vi "peg-in-hole Test with ref.vi"() -> ()   [LabVIEW 2013]
uses:
  Arm Globals.vi
  <vilib>/Utility/file.llb/Write To Spreadsheet File (DBL).vi
panel:
  in  "Pin Array":dbl[](array[numeric])
  in  "Save":bool
  in  "Peg Positions":i32[](array[numeric])
  out "Loops Remaining":i32=1
  out "Peg":i32=1
  out "Times":dbl[](array[numeric])=[14.65, 8.4, 8.4, 7.7, 7.75, 7.5, 8.1, 7.7, 8.4, 7.65, 7.65, 7.7, 8.35, 7.7, 32.2, 8.1, 8.25, 7.5, 7.8, 7.8, 7.7, 7.8500000000000005, 8.5, 7.4, 8.85, 8.05, 8.55, 7.5, 8.2, 7.8, 8.8, 7.55, 8.25, 7.3500000000000005, 8.85, 7.5, 8.65, 7.65, 8.950000000000001, 7.7, 7.5, 14.85, 7.6000000000000005, 7.6000000000000005, 9.05, 14.15, 15.200000000000001, 7.6000000000000005, 15.4, 7.5, 17.45, 7.5, 35.6, 7.75, 22.45, 7.45, 8.9, 7.75, 23.150000000000002, 7.95, 7.6000000000000005, 8.5, 8.9, 7.95, 8.2, 47.099000000000004, 21.150000000000002, 71.75, 9.0, 7.8500000000000005, 43.7, 16.1, 8.2, 8.1, 8.700000000000001, 16.2, 8.700000000000001, 7.7, 15.450000000000001, 7.3500000000000005, 7.8500000000000005, 7.55, 14.4, 7.4, 8.3, 7.6000000000000005, 14.4, 7.75, 8.3, 7.7, 8.25, 7.75, 8.0, 7.45, 14.3, 7.5, 8.2, 7.4, 7.7490000000000006, 7.8, 8.15, 7.5, 7.7, 7.7]
  out "Status":string="Test.4"
  in  "Stop":bool
  out "error out":errorcluster
  # "1\n2\n3\n4\n5\n6\n7"
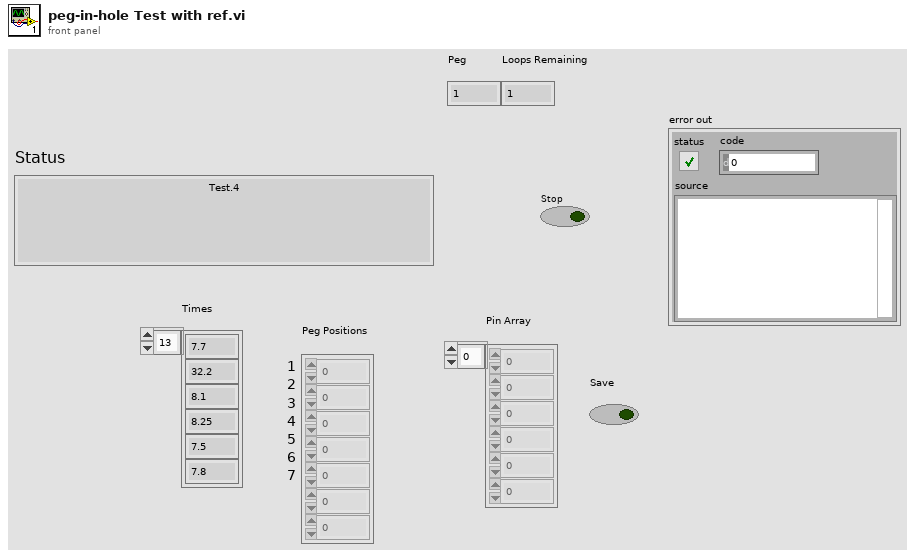
[diagram p1: front panel]
types:
  T1 = cluster{"X":dbl, "Y":dbl, "Z":dbl, "O":dbl, "A":dbl, "T":dbl}
  T2 = cluster{"X":dbl, "Y":dbl, "Z":dbl, "O":dbl, "A":dbl, "T":dbl}[]
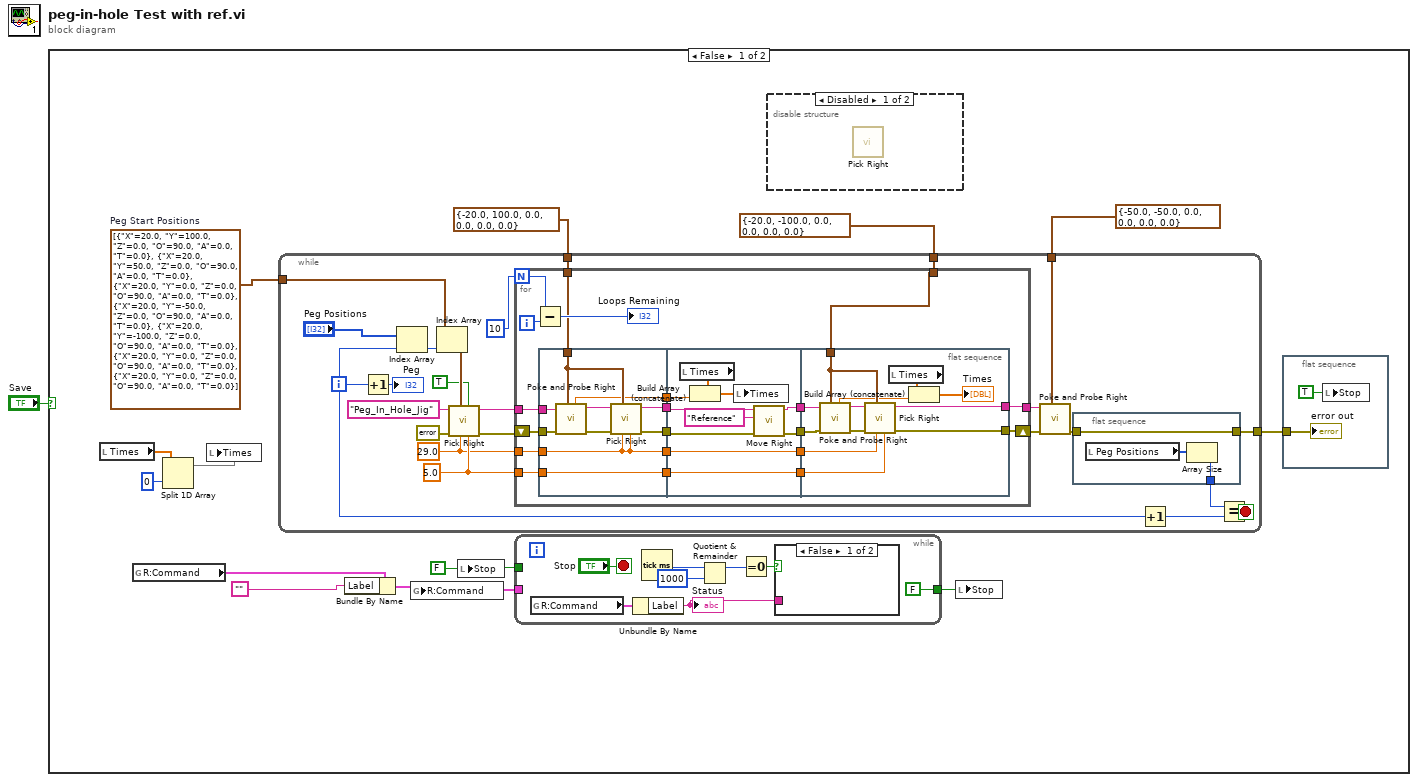
[diagram p0: block diagram]
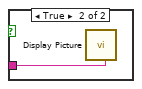
[diagram p3: hidden frame]
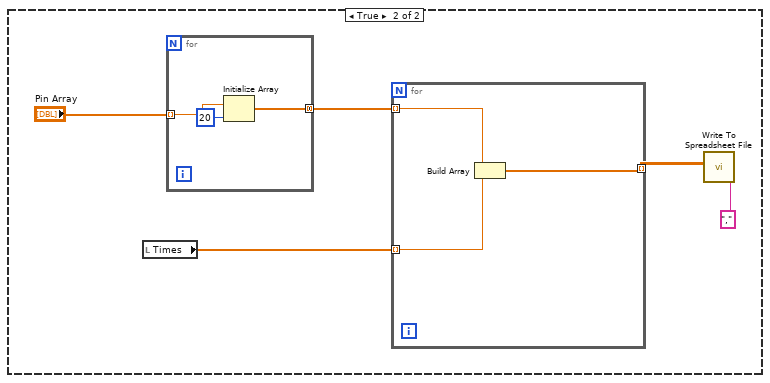
[diagram p4: hidden frame]
diagram:
  n1 = case shown="False" "Save" {
    frame False {
      w10 = FALSE ("Stop")
      w5 = T2 [{"X"=20.0, "Y"=100.0, "Z"=0.0, "O"=90.0, "A"=0.0, "T"=0.0}, {"X"=20.0, "Y"=50.0, "Z"=0.0, "O"=90.0, "A"=0.0, "T"=0.0}, {"X"=20.0, "Y"=0.0, "Z"=0.0, "O"=90.0, "A"=0.0, "T"=0.0}, {"X"=20.0, "Y"=-50.0, "Z"=0.0, "O"=90.0, "A"=0.0, "T"=0.0}, {"X"=20.0, "Y"=-100.0, "Z"=0.0, "O"=90.0, "A"=0.0, "T"=0.0}, {"X"=20.0, "Y"=0.0, "Z"=0.0, "O"=90.0, "A"=0.0, "T"=0.0}, {"X"=20.0, "Y"=0.0, "Z"=0.0, "O"=90.0, "A"=0.0, "T"=0.0}]  # Peg Start Positions
      n2 = local read "Times"() -> (w13:dbl[])
      n3 = global read "Arm Globals.vi" "R:Command"() -> (w6:cluster{"Label":string, "Angles":dbl[]})
      n4 = Split 1D Array(array=w13, index=0) -> (first subarray=w11:dbl[])  [unwired: 1 out]
      n5 = local write "Times"(w11) -> ()
      n6 = while {
        tunnel: [w21] -> w14
        tunnel: w5 -> [w34]
        tunnel: T1 {"X"=-20.0, "Y"=-100.0, "Z"=0.0, "O"=0.0, "A"=0.0, "T"=0.0} ("x") -> [w35]
        tunnel: T1 {"X"=-50.0, "Y"=-50.0, "Z"=0.0, "O"=0.0, "A"=0.0, "T"=0.0} ("x") -> [w36]
        tunnel: T1 {"X"=-20.0, "Y"=100.0, "Z"=0.0, "O"=0.0, "A"=0.0, "T"=0.0} ("x") -> [w29]
        i -> [w16]
        stop <- w26 stop-if-true
        w18 = sgl 5.0 ("Threshold")
        w17 = sgl 29.0 ("Target Position")
        n7 = Increment(x=w16) -> (x+1=→"Peg":i32)
        n8 = Index Array(array="Peg Positions", index=w16) -> (element=w32:i32)
        n9 = Index Array(array=w34, index=w32) -> (element=w33:T1)
        n10 = call "Pick Right.vi"("Threshold"=w18, "Pause on Miss?"=TRUE, "Target Position"=w17, "Pick"=w33, "error in"=errorcluster {"status"=FALSE, "code"=0, "source"=""}, "Location"="Peg_In_Hole_Jig") -> ("error out"=w31:errorcluster, "Location Out"=w24:string)  [unwired: 4 in]
        n11 = for {
          N: 10 -> [w61]
          shift-right: [w50] -> w30
          shift-left: w31 -> [w58]
          tunnel: w35 -> [w51]
          tunnel: w29 -> [w56]
          tunnel: w24 -> [w57]
          tunnel: [w49] -> w23
          tunnel: w18 -> [w45]
          tunnel: w17 -> [w42]
          i -> [w60]
          n12 = Subtract(x=w61, y=w60) -> (x-y=→"Loops Remaining":i32)
          n13 = flat-sequence {
            tunnel: w58 -> [w71]
            tunnel: w57 -> [w70]
            tunnel: w56 -> [w69]
            tunnel: [w67] -> w55
            tunnel: [w65] -> w54
            tunnel: [w64] -> w53
            tunnel: [w63] -> w46
            tunnel: w45 -> [w63]
            tunnel: [w62] -> w43
            tunnel: w42 -> [w62]
            tunnel: w55 -> [w77]
            tunnel: w54 -> [w80]
            tunnel: w53 -> [w76]
            tunnel: [w78] -> w52
            tunnel: [w75] -> w48
            tunnel: [w73] -> w47
            tunnel: w46 -> [w73]
            tunnel: [w72] -> w44
            tunnel: w43 -> [w72]
            tunnel: w52 -> [w92]
            tunnel: w51 -> [w89]
            tunnel: [w85] -> w50
            tunnel: [w84] -> w49
            tunnel: w48 -> [w93]
            tunnel: w47 -> [w83]
            tunnel: w44 -> [w82]
            frame #0 {
              n14 = call "Poke and Probe Right.vi"("Goal"=w69, "error in"=w71, "Location"=w70) -> ("error out"=w66:errorcluster, "Location Out"=w68:string, "time"=w65:dbl)  [unwired: 6 in]
              n15 = call "Pick Right.vi"("Threshold"=w62, "Target Position"=w62, "Pick"=w69, "error in"=w66, "Location"=w68) -> ("error out"=w67:errorcluster, "Location Out"=w64:string)  [unwired: 5 in]
            }
            frame #1 {
              n16 = local read "Times"() -> (w81:dbl[])
              n17 = Build Array (concatenate)(w81, w80) -> (w79:dbl[])
              n18 = local write "Times"(w79) -> ()
              n19 = call "Move Right.vi"("error in"=w77, "Mask"="Reference", "Location"=w76) -> ("error out"=w78:errorcluster, "Location Out"=w75:string)  [unwired: 4 in, 3 out]
            }
            frame #2 {
              n20 = call "Poke and Probe Right.vi"("Goal"=w89, "error in"=w92, "Location"=w93) -> ("error out"=w91:errorcluster, "Location Out"=w90:string, "time"=w86:dbl)  [unwired: 6 in]
              n21 = call "Pick Right.vi"("Threshold"=w83, "Target Position"=w82, "Pick"=w89, "error in"=w91, "Location"=w90) -> ("error out"=w85:errorcluster, "Location Out"=w84:string)  [unwired: 5 in]
              n22 = local read "Times"() -> (w88:dbl[])
              n23 = Build Array (concatenate)(w88, w86) -> (→"Times":dbl[])
            }
          }
        }
        n24 = call "Poke and Probe Right.vi"("Goal"=w36, "error in"=w30, "Location"=w23) -> ("error out"=w22:errorcluster)  [unwired: 6 in, 2 out]
        n25 = flat-sequence {
          tunnel: w22 -> [w41]
          tunnel: [w41] -> w21
          tunnel: [w39] -> w20
          frame #0 {
            n26 = local read "Peg Positions"() -> (w40:i32[])
            n27 = Array Size(array=w40) -> (size(s)=w39:i32)
          }
        }
        n28 = Increment(x=w16) -> (x+1=w15:i32)
        n29 = Equal?(x=w20, y=w15) -> (x = y?=w26:bool)
      }
      n30 = Bundle By Name(cluster=w6, "Label"="") -> (w8:cluster{"Label":string, "Angles":dbl[]})
      n31 = global write "Arm Globals.vi" "R:Command"(w8) -> ()
      n32 = local write "Stop"(w10) -> ()
      n33 = while {
        tunnel: w8 -> [_]
        tunnel: [FALSE] -> w9
        tunnel: w10 -> [_]
        stop <- "Stop" stop-if-true
        n34 = global read "Arm Globals.vi" "R:Command"() -> (w101:cluster{"Label":string, "Angles":dbl[]})
        n35 = Unbundle By Name(w101) -> ("Label"=w94:string)
        "Status" <- w94
        n36 = Tick Count (ms)() -> (millisecond timer value=w98:u32)
        n37 = Quotient & Remainder(x=w98, y=u32 1000) -> (x-y*floor(x/y)=w96:u32)  [unwired: 1 out]
        n38 = Equal To 0?(x=w96) -> (x = 0?=w95:bool)
        n39 = case shown="False" w95 {
          tunnel: w94 -> [_ w102]
          frame False {
          }
          frame True {
            n40 = call "Display Picture.vi"("Comment"=w102) -> ()  [unwired: 10 in, 1 out]
          }
        }
      }
      n41 = disable-structure shown="Disabled" {
        frame Disabled {
          n42 = call "Pick Right.vi"() -> ()  [unwired: 10 in, 2 out]
        }
        frame Enabled {
        }
      }
      n43 = local write "Stop"(w9) -> ()
      n44 = flat-sequence {
        tunnel: w14 -> [w104]
        frame #0 {
          n45 = local write "Stop"(TRUE ("Stop")) -> ()
          "error out" <- w104
        }
      }
    }
    frame True {
      n46 = local read "Times"() -> (w107:dbl[])
      n47 = for {
        tunnel: "Pin Array" -> [w115] mode=indexing
        tunnel: [w113] -> w108 mode=concatenating
        n48 = Initialize Array(w115, 20 ("dimension size")) -> (w113:dbl[])
      }
      n49 = for {
        tunnel: w108 -> [w112] mode=indexing
        tunnel: w107 -> [w111] mode=indexing
        tunnel: [w110] -> w106 mode=indexing
        n50 = Build Array(w112, w111) -> (w110:dbl[])
      }
      n51 = call-poly <vilib>:"Write To Spreadsheet File.vi"("delimiter (\\t)"="," ("delimiter (\\t)"), "2D data"=w106) -> ()  [unwired: 6 in, 1 out]
    }
  }
